vi "EEPROM_Format_Notes.vi"(8 "error in (no error)":errorcluster, 10 "EEPROM data":string[](array[string]), 11 "Notes reference":refnum<vi>) -> (0 "error out":errorcluster)   [LabVIEW 2010, in "lib1299.lvlib"]
uses:
  lib1299.lvlib
panel:
  in  "Notes Formatting Text":string[](array[string])=["Device: %s", "Board Version: %s", "Assembly Version: %s", "BOM Version: %s", "Assembly Date: %s"]
  # "(This is constant text)"
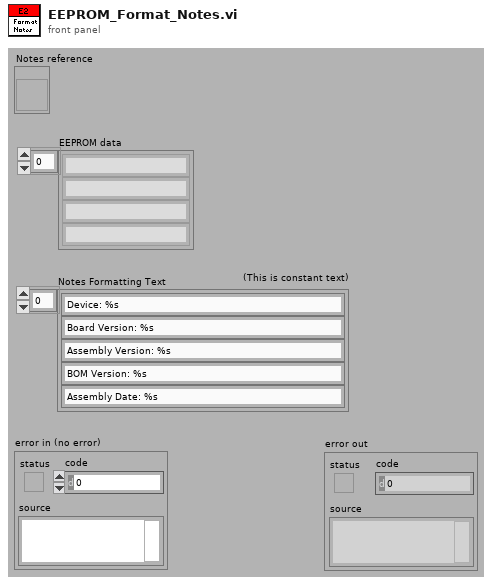
[diagram p1: front panel]
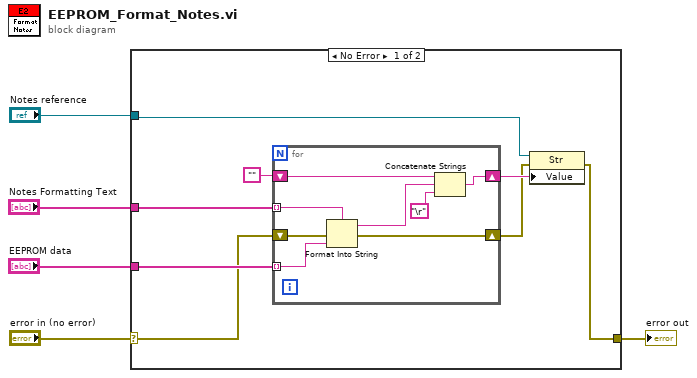
[diagram p0: block diagram]
diagram:
  n1 = case shown="No Error" "error in (no error)" {
    selector: "error in (no error)" -> [w8 w22]
    tunnel: [w9 w22] -> w4
    tunnel: "Notes reference" -> [w10 _]
    tunnel: "EEPROM data" -> [w13 _]
    tunnel: "Notes Formatting Text" -> [w11 _]
    frame No Error {
      n2 = for {
        tunnel: w13 -> [w21] mode=indexing
        shift-right: [w20] -> w12
        shift-left: "" -> [w19]
        tunnel: w11 -> [w17] mode=indexing
        shift-right: [w15] -> w7
        shift-left: w8 -> [w16]
        n3 = Format Into String(format string=w17, error in=w16, w21) -> (resulting string=w18:string, error out=w15:errorcluster)  [unwired: 1 in]
        n4 = Concatenate Strings(w19, w18, "\r") -> (w20:string)
      }
      n5 = property class="Str"(reference=w10, error in=w7, "Value"=w12) -> (error out=w9:errorcluster)  [unwired: 1 out]
    }
    frame Error {
    }
  }
  "error out" <- w4
